vi "FB Switch Bool Output Term No Var.vi"(8 "error in":errorcluster, 10 "invert":bool, 11 "data in":variant) -> (0 "error out":errorcluster, 3 "data out":variant)   [LabVIEW 2017]
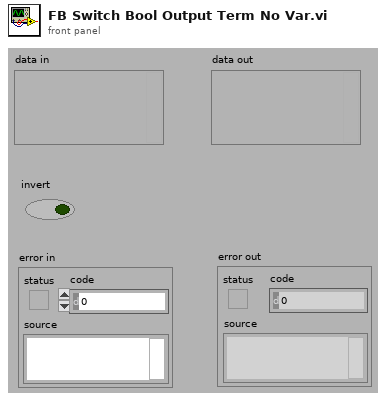
[diagram p1: front panel]
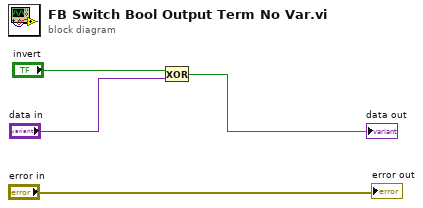
[diagram p0: block diagram]
diagram:
  n1 = Exclusive Or(1:"data in", 2:"invert") -> (0:→"data out":bool)
  "error out" <- "error in"
